vi "Time Estimate.vi"(8 "error in (no error)":errorcluster, 9 "expmode":i32, 10 "scantype":T1(ring), 11 "Varian Continuous.lvclass":refnum<class "Varian Continuous.lvclass">) -> (0 "error out":errorcluster, 1 "Time Estimate":string, 2 "time":dbl[unit], 3 "Varian Continuous.lvclass out":refnum<class "Varian Continuous.lvclass">)   [LabVIEW 2009, in "Varian Continuous.lvclass"]
doc: "(Dynamic) Return an estimate of the time remaining to scan over this Scanner's preconfigured Range."
uses:
  Varian Continuous.lvclass
  Scanner/Scanner.lvclass
  Varian Continuous.lvclass/Varian Continuous.ctl
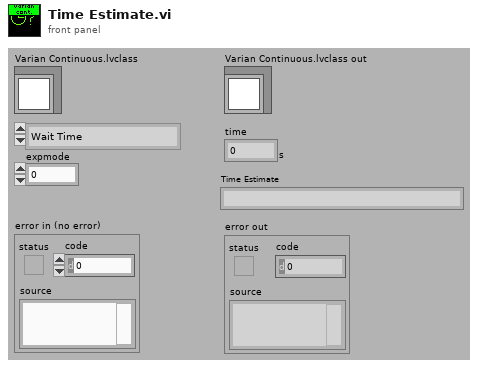
[diagram p1: front panel]
types:
  T1 = enum16{"Wait Time", "Pulse Width", "Wavelength", "Magnetic Field", "rf Scan"}
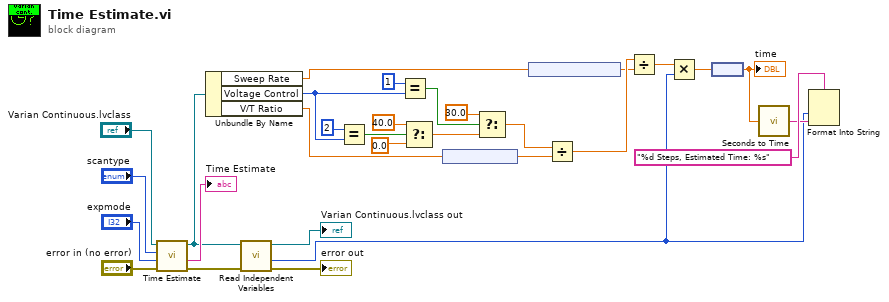
[diagram p0: block diagram]
diagram:
  n1 = call-parent "Time Estimate.vi"("error in (no error)"="error in (no error)", "expmode"="expmode", "scantype"="scantype", "Scanner.lvclass"="Varian Continuous.lvclass") -> ("error out"=w7:errorcluster, "Time Estimate"=→"Time Estimate":string, "Scanner.lvclass out"=w5:refnum<class "Varian Continuous.lvclass">)  [unwired: 4 in, 1 out]
  n2 = Unbundle By Name(w5) -> ("Sweep Rate"=w13:dbl[unit], "Voltage Control"=w22:u16, "V/T Ratio"=w16:dbl[unit])
  n3 = call-dynamic "Read Independent Variables.vi"("error in (no error)"=w7, "Scanner.lvclass in"=w5) -> ("error out"=→"error out":errorcluster, "size"=w1:i32, "Scanner.lvclass out"=→"Varian Continuous.lvclass out":refnum<class "Varian Continuous.lvclass">)  [unwired: 7 out]
  n4 = Equal?(x=2, y=w22) -> (x = y?=w20:bool)
  n5 = Equal?(x=1, y=w22) -> (x = y?=w25:bool)
  n6 = Select(t=40.0, s=w20, f=0.0) -> (s? t:f=w21:dbl)
  n7 = node(w16) -> (w11:dbl)
  n8 = Select(t=30.0, s=w25, f=w21) -> (s? t:f=w15:dbl)
  n9 = node(w13) -> (w12:dbl)
  n10 = Divide(x=w15, y=w11) -> (x/y=w14:dbl)
  n11 = Divide(x=w14, y=w12) -> (x/y=w4:dbl)
  n12 = Multiply(x=w4, y=w1) -> (x*y=w2:dbl)
  n13 = node(w2) -> (w3:dbl[unit])
  "time" <- w3
  n14 = call "Seconds to Time.vi"("Seconds"=w3) -> ("Time"=w9:string)
  n15 = Format Into String(format string="%d Steps, Estimated Time: %s", w1, w9) -> ()  [unwired: 2 in, 2 out]
